vi "readArduino.vi"() -> ()   [LabVIEW 2019]
uses:
  <vilib>/Instr/_visa.llb/VISA Configure Serial Port (Instr).vi
panel:
  out "Numeric":dbl
  out "Waveform Chart":dbl(graph)
  in  "stop":bool
  in  "byte count":u32
  in  "Enable Termination\nChar (T)":bool=TRUE
  in  "termination char\n(0xA = '\\n' = LF)":u8=10 format="%.0x"
  in  "flow control (0:none)":u16(ring) items=["None", "XON/XOFF", "RTS/CTS", "XON/XOFF & RTS/CTS", "DTR/DSR", "XON/XOFF & DTR/DSR"]
  in  "stop bits (10: 1 bit)":u16(ring)=10 items=["1.0"=10, "1.5"=15, "2.0"=20]
  in  "parity (0:none)":enum16{"None", "Odd", "Even", "Mark", "Space"}(ring)
  in  "data bits (8)":u16=8 min=5 max=8 step=1
  in  "baud rate (9600)":u32=9600
  in  "VISA resource name":refnum<visa-resource-name>
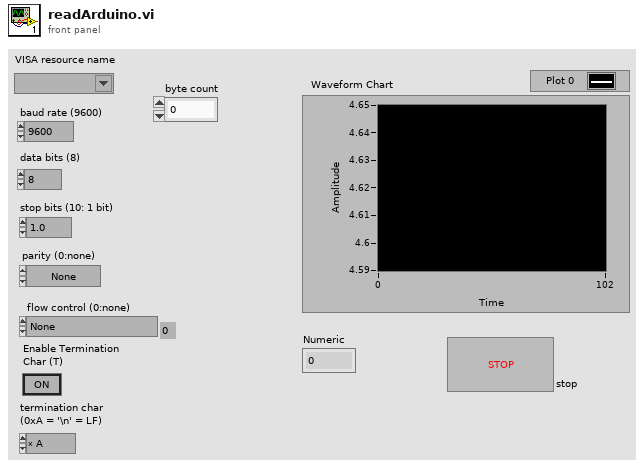
[diagram p1: front panel]
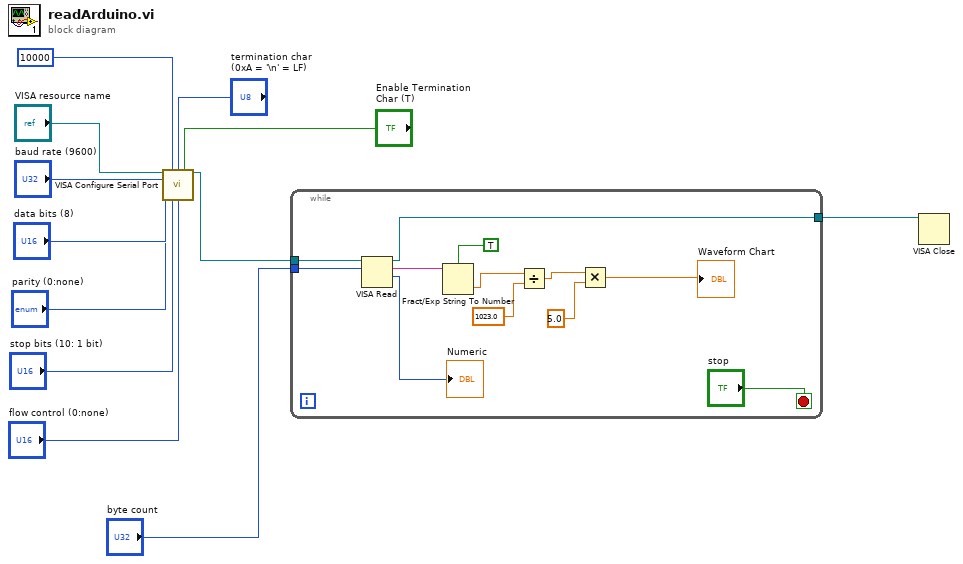
[diagram p0: block diagram]
diagram:
  n1 = call-poly "VISA Configure Serial Port"("VISA resource name"="VISA resource name", "timeout (10sec)"=u32 10000, "termination char\n(0xA = '\\n' = LF)"="termination char\n(0xA = '\\n' = LF)", "Enable Termination\nChar (T)"="Enable Termination\nChar (T)", "baud rate (9600)"="baud rate (9600)", "data bits (8)"="data bits (8)", "parity (0:none)"="parity (0:none)", "stop bits (10: 1 bit)"="stop bits (10: 1 bit)", "flow control (0:none)"="flow control (0:none)") -> ("VISA resource name out"=w3:refnum<visa-resource-name>)  [unwired: 5 in, 1 out]
  n2 = while {
    tunnel: w3 -> [w24]
    tunnel: "byte count" -> [w23]
    tunnel: [w13] -> w1
    stop <- "stop" stop-if-true
    n3 = VISA Read(VISA resource name=w24, byte count=w23) -> (VISA resource name out=w13:refnum<visa-resource-name>, read buffer=w21:string, return count=→"Numeric":u32)  [unwired: 1 in, 1 out]
    n4 = Fract/Exp String To Number(use system decimal point (T)=TRUE, string=w21) -> (number=w19:dbl)  [unwired: 2 in, 1 out]
    n5 = Divide(x=w19, y=1023.0) -> (x/y=w17:dbl)
    n6 = Multiply(x=w17, y=5.0) -> (x*y=→"Waveform Chart":dbl)
  }
  n7 = VISA Close(VISA resource name=w1) -> ()  [unwired: 1 in, 1 out]
